vi "Audio_Transformation_Setted_Frequency_v011.vi"() -> ()   [LabVIEW 2019]
uses:
  <vilib>/sound2/lvsound2.llb/Sound Data Format.ctl
  <vilib>/sound2/lvsound2.llb/Sound Input Read (DBL).vi
  <vilib>/addons/Time Frequency Analysis/Transform.llb/TFA Online Gabor Transform (Real).vi
  <vilib>/addons/_Advanced Signal Processing/NI_AdvSigProcTFA.lvlib
panel:
  out "u(t)":T1(graph)
  out "V(t)":T1(graph)
  out "Noise Speech":dbl[](graph)
  in  "Neuron Type":T2(ring)=enum."Phasic Spiking (PS)"
  out "max index(es)":i32
  out "max value":dbl
  out "Waveform Graph":dbl[](graph)
  out "Magnitude of Gabor Coefficients":dbl[][](graph)
  in  "Stop":bool
  # "Step two : Graph of the amplitude of the Gabor coefficient of the different bins"
  # "Step three : Spike Response of the neurons"
  # "Step one: Sound recorded from the computer"
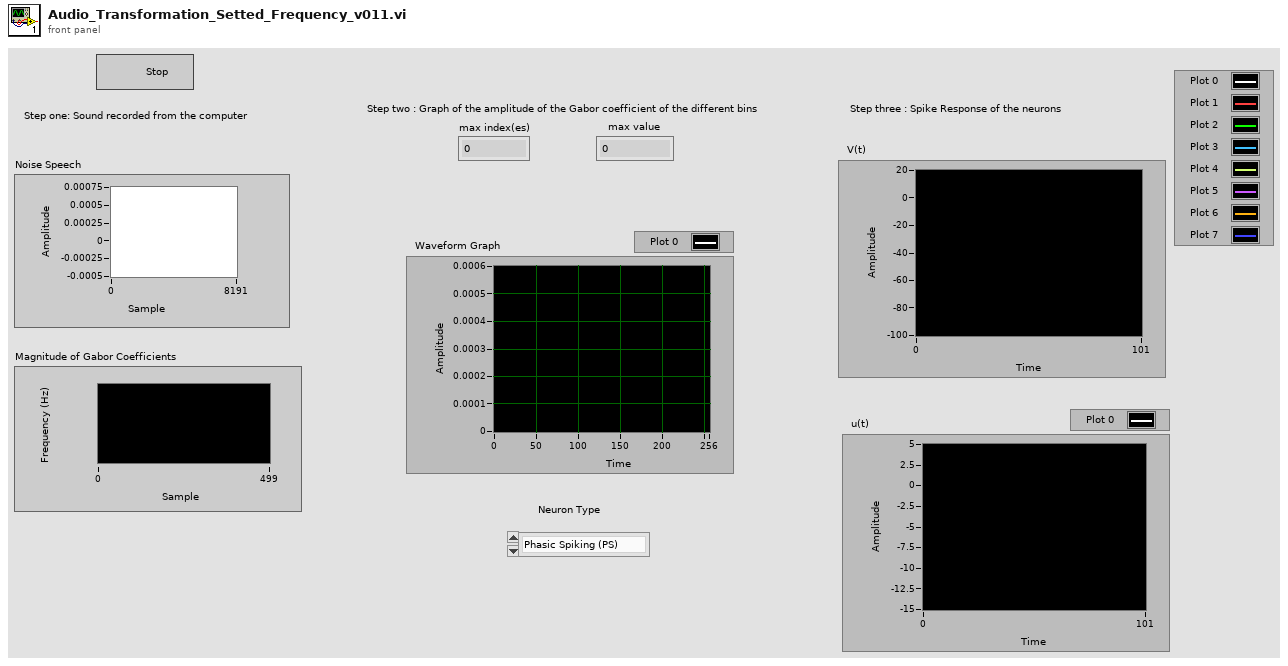
[diagram p1: front panel]
types:
  T1 = cluster{"[0]":dbl, "[1]":dbl, "[2]":dbl, "[3]":dbl, "[4]":dbl, "[5]":dbl, "[6]":dbl, "[7]":dbl}
  T2 = enum16{"Regular Spiking (RS)", "Intrinsically Bursting (IB)", "Chattering (CH)", "Fast Spiking (FS)", "Thalamo-Cortical 1 (TC1)", "Thalamo-Cortical 2 (TC2)", "Resonator (RZ)", "Low-Threshold Spiking (LTS)", "Phasic Spiking (PS)"}
  T3 = typedef "Sound Data Format.ctl" = cluster{"sample rate (S/s)":dbl, "number of channels":i32, "bits per sample":i32}
  T4 = cluster{"analysis window":dbl[], "dM (time steps)":i32, "N (frequency bins)":i32}
  T5 = typedef "Sound Input Task ID.ctl" = u32
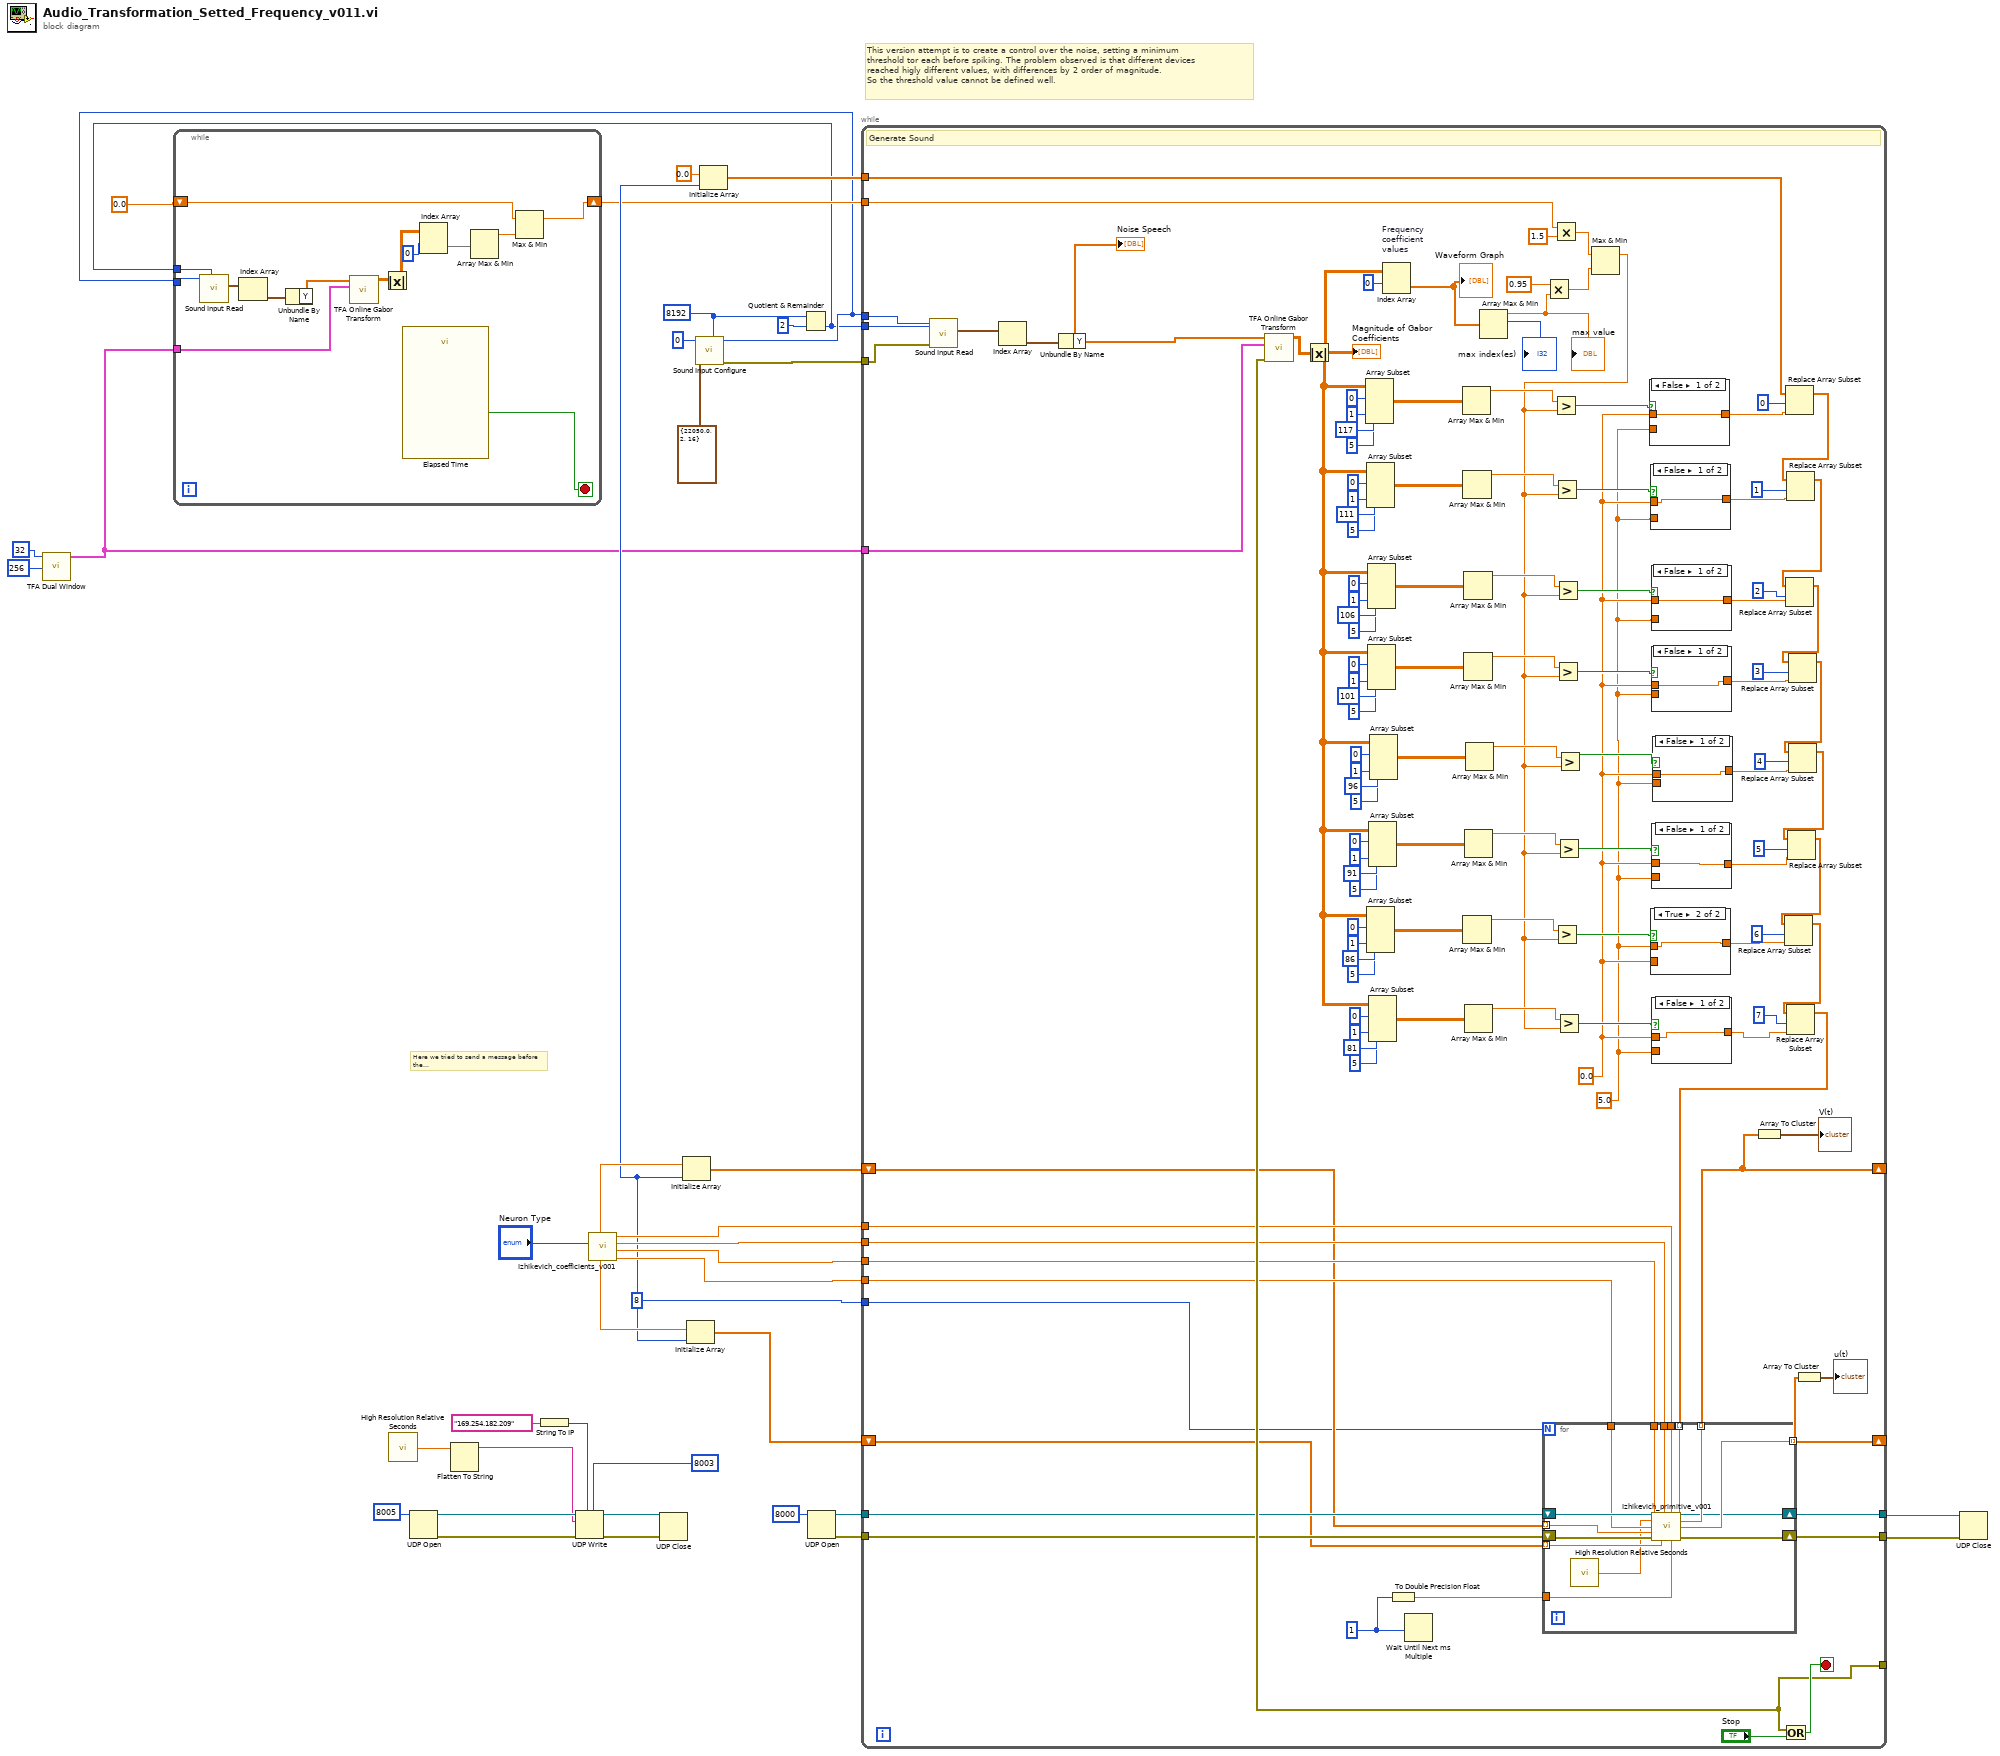
[diagram p0: block diagram]
diagram:
  w21 = 8
  w28 = 8192 ("number of samples/ch")
  # "Here we tried to send a message before the\nspiking session to coordinate the comunication"
  # "This version attempt is to create a control over the noise, setting a minimum\nthreshold tor each before spiking. The problem observed is that different devices\nreached higly different values, with differences by 2 order of magnitude.\nSo the threshold value cannot be defined well."
  n1 = call <vilib>:"TFA Dual Window.vi"("N (frequency bins)"=256, "dM (time steps)"=32) -> ("analysis info"=w18:T4)  [unwired: 7 in, 2 out]
  n2 = call <vilib>:"High Resolution Relative Seconds.vi"() -> ("relative seconds"=w6:dbl)
  n3 = UDP Open(11:u16 8005 ("port")) -> (port=w12:refnum<k16>, 0:w11:errorcluster)  [unwired: 4 in, 1 out]
  n4 = Flatten To String(anything=w6) -> (data string=w7:string)  [unwired: 3 in, 2 out]
  n5 = String To IP(1:"169.254.182.209" ("name")) -> (0:w9:u32)
  n6 = UDP Write(address=w9, port or service name=u16 8003, connection ID=w12, data in=w7, 8:w11) -> (error out=w2:errorcluster, 3:w3:refnum<k16>)  [unwired: 1 in]
  n7 = call "Izhikevich_coefficients_v001.vi"("Neuron Type"="Neuron Type") -> ("d"=w33:dbl, "c"=w34:dbl, "b"=w35:dbl, "a"=w36:dbl, "u0"=w23:dbl, "v0"=w25:dbl)  [unwired: 3 in]
  n8 = UDP Close(connection ID=w3, 8:w2) -> ()  [unwired: 2 out]
  n9 = Initialize Array(w25, w21) -> (w24:dbl[])
  n10 = Initialize Array(w23, w21) -> (w22:dbl[])
  n11 = call <vilib>:"Sound Input Configure.vi"("number of samples/ch"=w28, "sound format"=T3 {"sample rate (S/s)"=22050.0, "number of channels"=2, "bits per sample"=16}, "device ID"=u32 0) -> ("error out"=w26:errorcluster, "task ID"=w15:T5)  [unwired: 7 in]
  n12 = Initialize Array(0.0 ("element"), w21) -> (w19:dbl[])
  n13 = Quotient & Remainder(x=w28, y=2) -> (floor(x/y)=w14:i32)  [unwired: 1 out]
  n14 = while {
    tunnel: w18 -> [w51]
    shift-right: [w43] -> w16
    shift-left: 0.0 -> [w44]
    tunnel: w15 -> [w41]
    tunnel: w14 -> [w40]
    stop <- w42 stop-if-true
    n15 = call-poly <vilib>:"Sound Input Read.vi"("number of samples/ch"=w40, "task ID"=w41) -> ("data"=w52:waveform(dbl)[])  [unwired: 7 in, 2 out]
    n16 = Index Array(array=w52) -> (element=w53:waveform(dbl))  [unwired: 1 in]
    n17 = Unbundle By Name(w53) -> ("Y"=w50:dbl[])
    n18 = call-poly <vilib>:"TFA Online Gabor Transform.vi"("transform info"=w51, "signal"=w50) -> ("Gabor coef"=w49:cdb[][])  [unwired: 7 in, 2 out]
    n19 = Absolute Value(x=w49) -> (abs(x)=w47:dbl[][])
    n20 = call "Elapsed Time"() -> ("Time has Elapsed"=w42:bool)  [unwired: 12 in, 7 out]
    n21 = Index Array(array=w47, index (row)=0) -> (element=w46:dbl[])  [unwired: 1 in]
    n22 = Array Max & Min(array=w46) -> (max value=w45:dbl)  [unwired: 3 out]
    n23 = Max & Min(x=w44, y=w45) -> (max(x,y)=w43:dbl)  [unwired: 1 out]
  }
  n24 = UDP Open(11:u16 8000 ("port")) -> (port=w5:refnum<k16>, 0:w4:errorcluster)  [unwired: 4 in, 1 out]
  n25 = while {
    tunnel: [w168] -> _
    tunnel: w18 -> [w173]
    shift-right: [w67] -> _
    shift-left: w24 -> [w157]
    shift-right: [w65] -> _
    shift-left: w22 -> [w156]
    tunnel: w36 -> [w167]
    tunnel: w35 -> [w166]
    tunnel: w34 -> [w164]
    tunnel: w33 -> [w163]
    tunnel: w5 -> [w165]
    tunnel: w4 -> [w162]
    tunnel: [w159] -> w32
    tunnel: [w158] -> w31
    tunnel: w15 -> [w154]
    tunnel: w26 -> [w153]
    tunnel: w14 -> [w155]
    tunnel: w21 -> [w149]
    tunnel: w19 -> [w121]
    tunnel: w16 -> [w61]
    stop <- w174 stop-if-true
    w55 = 5.0
    w56 = 0.0
    w161 = u32 1 ("millisecond multiple")
    # "Generate Sound"
    n26 = call-poly <vilib>:"Sound Input Read.vi"("number of samples/ch"=w155, "error in (no error)"=w153, "task ID"=w154) -> ("data"=w151:waveform(dbl)[])  [unwired: 6 in, 2 out]
    n27 = Index Array(array=w151) -> (element=w152:waveform(dbl))  [unwired: 1 in]
    n28 = Unbundle By Name(w152) -> ("Y"=w150:dbl[])
    "Noise Speech" <- w150
    n29 = call-poly <vilib>:"TFA Online Gabor Transform.vi"("transform info"=w173, "signal"=w150) -> ("error out"=w168:errorcluster, "Gabor coef"=w172:cdb[][])  [unwired: 7 in, 1 out]
    n30 = Absolute Value(x=w172) -> (abs(x)=w70:dbl[][])
    "Magnitude of Gabor Coefficients" <- w70
    n31 = Array Subset(array=w70, index (row)=0 ("index"), length (row)=1 ("length"), index (col)=117 ("index"), length (col)=5 ("length")) -> (w144:dbl[][])
    n32 = Array Subset(array=w70, index (row)=0 ("index"), length (row)=1 ("length"), index (col)=111 ("index"), length (col)=5 ("length")) -> (w137:dbl[][])
    n33 = Array Subset(array=w70, index (row)=0 ("index"), length (row)=1 ("length"), index (col)=86 ("index"), length (col)=5 ("length")) -> (w84:dbl[][])
    n34 = Array Subset(array=w70, index (row)=0 ("index"), length (row)=1 ("length"), index (col)=106 ("index"), length (col)=5 ("length")) -> (w126:dbl[][])
    n35 = Array Subset(array=w70, index (row)=0 ("index"), length (row)=1 ("length"), index (col)=101 ("index"), length (col)=5 ("length")) -> (w114:dbl[][])
    n36 = Array Subset(array=w70, index (row)=0 ("index"), length (row)=1 ("length"), index (col)=91 ("index"), length (col)=5 ("length")) -> (w94:dbl[][])
    n37 = Array Subset(array=w70, index (row)=0 ("index"), length (row)=1 ("length"), index (col)=81 ("index"), length (col)=5 ("length")) -> (w74:dbl[][])
    n38 = Array Subset(array=w70, index (row)=0 ("index"), length (row)=1 ("length"), index (col)=96 ("index"), length (col)=5 ("length")) -> (w104:dbl[][])
    n39 = Index Array "Frequency \ncoefficient \nvalues"(array=w70, index (row)=0) -> (element=w170:dbl[])  [unwired: 1 in]
    "Waveform Graph" <- w170
    n40 = To Double Precision Float(number=w161) -> (double precision float=w160:dbl)
    n41 = Wait Until Next ms Multiple(millisecond multiple=w161) -> ()  [unwired: 1 out]
    n42 = Array Max & Min(array=w144) -> (max value=w143:dbl)  [unwired: 3 out]
    n43 = Array Max & Min(array=w137) -> (max value=w136:dbl)  [unwired: 3 out]
    n44 = Array Max & Min(array=w84) -> (max value=w83:dbl)  [unwired: 3 out]
    n45 = Array Max & Min(array=w126) -> (max value=w125:dbl)  [unwired: 3 out]
    n46 = Array Max & Min(array=w114) -> (max value=w113:dbl)  [unwired: 3 out]
    n47 = Array Max & Min(array=w94) -> (max value=w93:dbl)  [unwired: 3 out]
    n48 = Array Max & Min(array=w74) -> (max value=w73:dbl)  [unwired: 3 out]
    n49 = Array Max & Min(array=w104) -> (max value=w103:dbl)  [unwired: 3 out]
    n50 = Array Max & Min(array=w170) -> (max value=w58:dbl, max index (indices)=→"max index(es)":i32)  [unwired: 2 out]
    "max value" <- w58
    n51 = Multiply(x=0.95 ("y"), y=w58) -> (x*y=w59:dbl)
    n52 = Multiply(x=w61, y=1.5) -> (x*y=w60:dbl)
    n53 = Max & Min(x=w60, y=w59) -> (max(x,y)=w63:dbl)  [unwired: 1 out]
    n54 = Greater?(x=w143, y=w63) -> (0:w142:bool)
    n55 = Greater?(x=w136, y=w63) -> (0:w135:bool)
    n56 = Greater?(x=w83, y=w63) -> (0:w82:bool)
    n57 = Greater?(x=w125, y=w63) -> (0:w124:bool)
    n58 = Greater?(x=w113, y=w63) -> (0:w112:bool)
    n59 = Greater?(x=w93, y=w63) -> (0:w92:bool)
    n60 = Greater?(x=w73, y=w63) -> (0:w72:bool)
    n61 = Greater?(x=w103, y=w63) -> (0:w102:bool)
    n62 = case shown="False" w142 {
      tunnel: [w190 w191] -> w134
      tunnel: w56 -> [w190 _]
      tunnel: w55 -> [_ w191]
      frame False {
      }
      frame True {
      }
    }
    n63 = case shown="False" w135 {
      tunnel: [w188 w189] -> w131
      tunnel: w56 -> [w188 _]
      tunnel: w55 -> [_ w189]
      frame False {
      }
      frame True {
      }
    }
    n64 = case shown="True" w82 {
      tunnel: [w178 w179] -> w80
      tunnel: w56 -> [w178 _]
      tunnel: w55 -> [_ w179]
      frame False {
      }
      frame True {
      }
    }
    n65 = case shown="False" w124 {
      tunnel: [w186 w187] -> w122
      tunnel: w56 -> [w186 _]
      tunnel: w55 -> [_ w187]
      frame False {
      }
      frame True {
      }
    }
    n66 = case shown="False" w112 {
      tunnel: [w184 w185] -> w110
      tunnel: w56 -> [w184 _]
      tunnel: w55 -> [_ w185]
      frame False {
      }
      frame True {
      }
    }
    n67 = case shown="False" w92 {
      tunnel: [w180 w181] -> w90
      tunnel: w56 -> [w180 _]
      tunnel: w55 -> [_ w181]
      frame False {
      }
      frame True {
      }
    }
    n68 = case shown="False" w72 {
      tunnel: [w176 w177] -> w54
      tunnel: w56 -> [w176 _]
      tunnel: w55 -> [_ w177]
      frame False {
      }
      frame True {
      }
    }
    n69 = case shown="False" w102 {
      tunnel: [w182 w183] -> w100
      tunnel: w56 -> [w182 _]
      tunnel: w55 -> [_ w183]
      frame False {
      }
      frame True {
      }
    }
    n70 = Or(x=w168, y="Stop") -> (x .or. y?=w174:bool)
    n71 = Replace Array Subset(array=w121, new element=w134, index=0) -> (w120:dbl[])
    n72 = Replace Array Subset(array=w120, new element=w131, index=1) -> (w119:dbl[])
    n73 = Replace Array Subset(array=w119, new element=w122, index=2) -> (w109:dbl[])
    n74 = Replace Array Subset(array=w109, new element=w110, index=3) -> (w99:dbl[])
    n75 = Replace Array Subset(array=w99, new element=w100, index=4) -> (w89:dbl[])
    n76 = Replace Array Subset(array=w89, new element=w90, index=5) -> (w79:dbl[])
    n77 = Replace Array Subset(array=w79, new element=w80, index=6) -> (w69:dbl[])
    n78 = Replace Array Subset(array=w69, new element=w54, index=7) -> (w68:dbl[])
    n79 = for {
      N: w149 -> [_]
      tunnel: w167 -> [w206]
      tunnel: w166 -> [w205]
      tunnel: w164 -> [w203]
      tunnel: w163 -> [w202]
      tunnel: w160 -> [w200]
      tunnel: [w199] -> w67 mode=indexing
      tunnel: [w198] -> w65 mode=indexing
      tunnel: w157 -> [w195] mode=indexing
      tunnel: w156 -> [w194] mode=indexing
      shift-right: [w196] -> w158
      shift-left: w165 -> [w204]
      shift-right: [w197] -> w159
      shift-left: w162 -> [w201]
      tunnel: w68 -> [w193] mode=indexing
      n80 = call <vilib>:"High Resolution Relative Seconds.vi"() -> ("relative seconds"=w192:dbl)
      n81 = call "Izhikevich_primitive_v001.vi"("UDP Network Connection in"=w204, "b"=w205, "a"=w206, "I"=w193, "c"=w203, "d"=w202, "v(t)"=w195, "Neuron ID"=w192, "error in (no error)"=w201, "u(t)"=w194, "dt"=w200) -> ("UDP Network Connection out"=w196:refnum<k16>, "v(t+dt)"=w199:dbl, "u(t+dt)"=w198:dbl, "error out"=w197:errorcluster)  [unwired: 1 in]
    }
    n82 = Array To Cluster(array=w67) -> (cluster=→"V(t)":T1)
    n83 = Array To Cluster(array=w65) -> (cluster=→"u(t)":T1)
  }
  n84 = UDP Close(connection ID=w31, 8:w32) -> ()  [unwired: 2 out]
